vi "Unpack Transfer Configurations.vi"(8 "error in":errorcluster, 11 "Group Configurations":refnum<class "Group Configuration.lvclass">[](array[class])) -> (0 "error out":errorcluster, 1 "Labeled RX Transfer Configurations":T2(array[cluster]), 2 "Labeled TX Transfer Configurations":T2(array[cluster]))   [LabVIEW 2020, in "RDMA.lvlib" / "RDMA Transceiver.lvclass"]
doc: "Unpacks all Transfer Configuration objects from an array of group configurations, bundles the transfer configurations with their group and tranfer IDs, and returns these bundles in two seperate arrays: one array for TX transfers and one for RX transfers."
uses:
  RDMA Transceiver.lvclass
  DSF Core.lvlibp/Classes/Configuration/Core/Group/Group Configuration.lvclass
  DSF Core.lvlibp/Classes/Configuration/Core/Transfer/Transfer Configuration.lvclass
  Transfer Parameters.ctl
  DSF Core.lvlibp/Typedefs/DSF Direction.ctl
  DSF Core.lvlibp
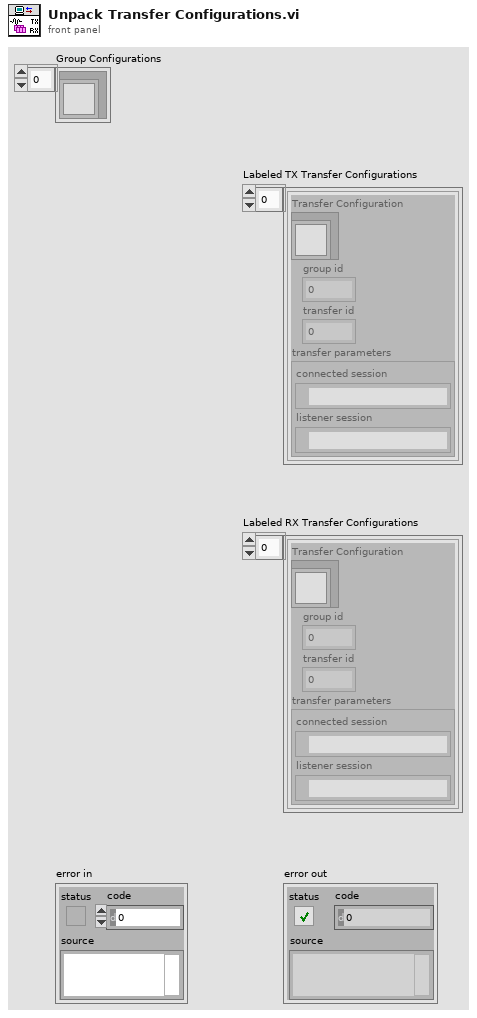
[diagram p1: front panel]
types:
  T1 = typedef "RDMA.lvlib/RDMA Transceiver.lvclass/Transfer Parameters.ctl" = cluster{"connected session":refnum<k21>, "listener session":refnum<k21>}
  T2 = cluster{"Transfer Configuration":refnum<class "Transfer Configuration.lvclass">, "group id":i32, "transfer id":i32, "transfer parameters":T1}[]
  T3 = typedef "DSF Core.lvlibp/DSF Direction.ctl" = enum8{"Tx", "Rx"}
  T4 = cluster{"Transfer Configuration":refnum<class "Transfer Configuration.lvclass">, "group id":i32, "transfer id":i32, "transfer parameters":T1}
  T5 = typedef "DSF Core.lvlibp/Group Configuration.lvclass/Core Group Configuration.ctl" = cluster{"name":string, "direction":T3, "cycle timing":T6, "timeout behavior":T7, "enable conversion":bool}
  T6 = typedef "DSF Core.lvlibp/DSF Timing Info.ctl" = cluster{"priority":u64, "decimation":u64, "offset":u64}
  T7 = typedef "DSF Core.lvlibp/DSF Timeout Behavior.ctl" = enum8{"Increment Late Count", "Throw Error"}
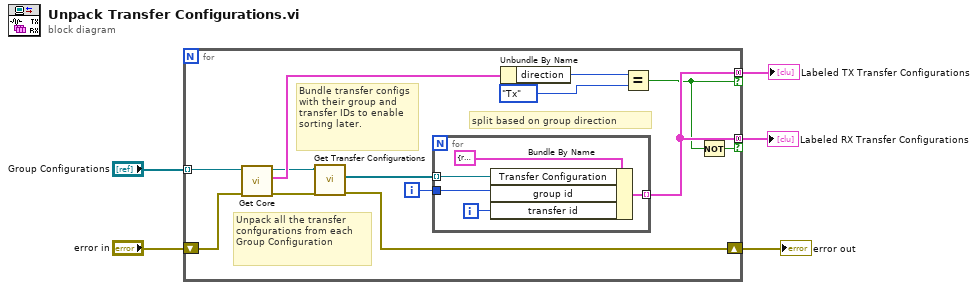
[diagram p0: block diagram]
diagram:
  n1 = for {
    tunnel: "Group Configurations" -> [w15] mode=indexing
    tunnel: [w12] -> w3 mode=concatenating if=w11
    shift-right: [w16] -> w4
    shift-left: "error in" -> [w8]
    tunnel: [w12] -> w2 mode=concatenating if=w10
    i -> [w17]
    # "split based on group direction"
    # "Unpack all the transfer confgurations from each Group Configuration"
    # "Bundle transfer configs with their group and transfer IDs to enable sorting later."
    n2 = call "Get Core.vi"("error in (no error)"=w8, "Group Configuration in"=w15) -> ("error out"=w9:errorcluster, "core"=w14:T5, "Group Configuration out"=w7:refnum<class "Group Configuration.lvclass">)  [unwired: 7 in]
    n3 = call "Get Transfer Configurations.vi"("error in (no error)"=w9, "Group Configuration in"=w7) -> ("error out"=w16:errorcluster, "Transfer Configurations"=w18:refnum<class "Transfer Configuration.lvclass">[])  [unwired: 7 in, 1 out]
    n4 = for {
      tunnel: w18 -> [w22] mode=indexing
      tunnel: w17 -> [w20]
      tunnel: [w19] -> w12 mode=indexing
      i -> [w21]
      n5 = Bundle By Name(cluster=T4 {"Transfer Configuration"=refnum, "group id"=0, "transfer id"=0, "transfer parameters"={"connected session"="", "listener session"=""}}, "Transfer Configuration"=w22, "group id"=w20, "transfer id"=w21) -> (w19:T4)
    }
    n6 = Unbundle By Name(w14) -> ("direction"=w13:T3)
    n7 = Equal?(x=w13, y=DSF_Direction."Tx") -> (x = y?=w11:bool)
    n8 = Not(x=w11) -> (.not. x?=w10:bool)
  }
  "error out" <- w4
  "Labeled TX Transfer Configurations" <- w3
  "Labeled RX Transfer Configurations" <- w2
